vi "Configure Trigger (USB).vi"(6 "Trigger Type (0: Start of Packet )":i32(ring) items=["Start of Packet ", "End of Packet", "Enter Suspend", "Exit Suspend", "Reset"], 7 "Speed (0: Low Speed)":i32(ring) items=["Low Speed", "Full Speed"], 8 "error in (no error)":errorcluster, 9 "D+ Source (1: Channel 2)":i32(ring)=1 items=["Channel 1"=0, "Channel 2"=1, "Channel 3"=2, "Channel 4"=3, "D0"=13, "D1"=14, "D2"=15, "D3"=16, "D4"=17, "D5"=18, "D6"=19, "D7"=20, "D8"=21, "D9"=22, "D10"=23, "D11"=24, "D12"=25, "D13"=26, "D14"=27, "D15"=28, "External"=29], 10 "D- Source (0: Channel 1)":i32(ring) items=["Channel 1"=0, "Channel 2"=1, "Channel 3"=2, "Channel 4"=3, "D0"=13, "D1"=14, "D2"=15, "D3"=16, "D4"=17, "D5"=18, "D6"=19, "D7"=20, "D8"=21, "D9"=22, "D10"=23, "D11"=24, "D12"=25, "D13"=26, "D14"=27, "D15"=28, "External"=29], 11 "VISA resource name":refnum<visa-resource-name>) -> (0 "error out":errorcluster, 3 "VISA resource name out":refnum<visa-resource-name>)   [LabVIEW 2015, in "Agilent 2000 3000 X-Series.lvlib"]
doc: "Configures the USB trigger mode.\n\n<B>Note(s):</B>\nThis VI is not applicable for Agilent InfiniiVision 4000 X-Series Oscilloscopes."
uses:
  Agilent 2000 3000 X-Series.lvlib
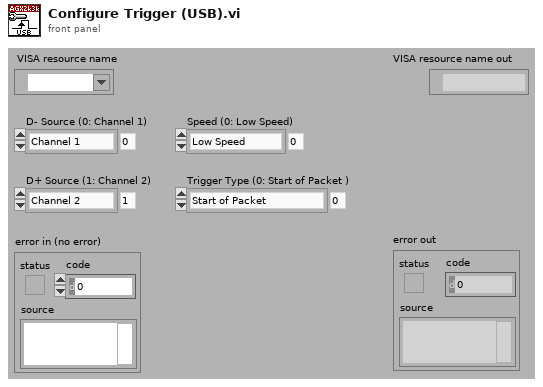
[diagram p1: front panel]
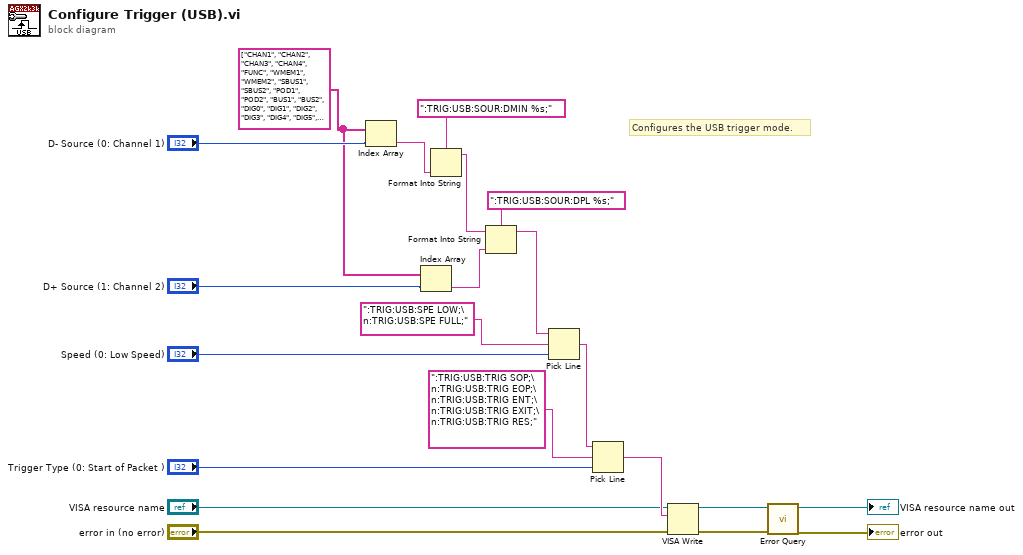
[diagram p0: block diagram]
diagram:
  w3 = string[] ["CHAN1", "CHAN2", "CHAN3", "CHAN4", "FUNC", "WMEM1", "WMEM2", "SBUS1", "SBUS2", "POD1", "POD2", "BUS1", "BUS2", "DIG0", "DIG1", "DIG2", "DIG3", "DIG4", "DIG5", "DIG6", "DIG7", "DIG8", "DIG9", "DIG10", "DIG11", "DIG12", "DIG13", "DIG14", "DIG15", "EXT", "LINE", "WGEN"]
  # "Configures the USB trigger mode."
  n1 = Index Array(array=w3, index="D- Source (0: Channel 1)") -> (element=w4:string)
  n2 = Index Array(array=w3, index="D+ Source (1: Channel 2)") -> (element=w2:string)
  n3 = Format Into String(format string=":TRIG:USB:SOUR:DMIN %s;", w4) -> (resulting string=w7:string)  [unwired: 2 in, 1 out]
  n4 = Format Into String(format string=":TRIG:USB:SOUR:DPL %s;", initial string=w7, w2) -> (resulting string=w6:string)  [unwired: 1 in, 1 out]
  n5 = Pick Line(string ("")=w6, multi-line string=":TRIG:USB:SPE LOW;\n:TRIG:USB:SPE FULL;", line index="Speed (0: Low Speed)") -> (output string=w17:string)
  n6 = Pick Line(string ("")=w17, multi-line string=":TRIG:USB:TRIG SOP;\n:TRIG:USB:TRIG EOP;\n:TRIG:USB:TRIG ENT;\n:TRIG:USB:TRIG EXIT;\n:TRIG:USB:TRIG RES;", line index="Trigger Type (0: Start of Packet )") -> (output string=w16:string)
  n7 = VISA Write(VISA resource name="VISA resource name", write buffer=w16, error in (no error)="error in (no error)") -> (VISA resource name out=w13:refnum<visa-resource-name>, error out=w12:errorcluster)  [unwired: 1 out]
  n8 = call "Error Query.vi"("error in (no error)"=w12, "VISA resource name"=w13) -> ("error out"=→"error out":errorcluster, "VISA resource name out"=→"VISA resource name out":refnum<visa-resource-name>)  [unwired: 8 out]
